vi "Main.vi"(8 "error in (no error)":errorcluster, 11 "ModuleAdmin":refnum<class "ModuleAdmin.lvclass">) -> ()   [LabVIEW 2018, in "SyncModule.lvlib"]
uses:
  SyncModule.lvlib
  <userlib>/NIST/ModuleAdminLib/ModuleAdmin/ModuleAdmin.lvclass
  C:/Program Files (x86)/National Instruments/LabVIEW 2018/user.lib/NIST/ModuleAdminLib/ModuleAdminBase/ModuleAdminBase.lvclass
  SyncPlugins/SyncPluginBase/SyncPluginBase.lvclass
  C:/Program Files (x86)/National Instruments/LabVIEW 2018/user.lib/NIST/BaseClasses/BasePlugin_class/BasePlugin.lvclass
  PublicAPI/Arguments/Requests/clStopArgument.ctl
  SyncPlugins/SyncPluginBase/SyncPluginBase.lvclass/SyncPluginBase.ctl
  <userlib>/NIST/BaseClasses/BasePlugin_class/BasePlugin.lvclass/BasePlugin.ctl
  <userlib>/NIST/ModuleAdminLib/ModuleAdmin/ModuleAdmin.lvclass/ModuleAdmin.ctl
  SyncPlugins/SyncPluginBase/Typedefs/clEnaTrigTmstmp.ctl
  SyncPlugins/SyncPluginBase/Typedefs/clGetTrigTmstmp.ctl
  SyncPlugins/SyncPluginBase/Typedefs/clTimedTrigger.ctl
  <vilib>/Utility/error.llb/DialogType.ctl
  SyncPlugins/SyncPluginBase/Accessors/Read PPSTime.vi
  <userlib>/NIST/BaseClasses/BasePlugin_class/Accessors/Read PluginIniFilePath.vi
  <userlib>/NIST/ModuleAdminLib/ModuleAdmin/Accessors/Read ShowPanel_.vi
  <userlib>/NIST/ModuleAdminLib/ModuleAdmin/Accessors/Write ShowPanel_.vi
  <userlib>/NIST/BaseClasses/BasePlugin_class/Accessors/Write PluginIniFilePath.vi
  SyncPlugins/SyncPluginBase/Accessors/Write LostLock.vi
  <userlib>/NIST/ModuleAdminLib/ModuleAdmin/Accessors/Read CloneRegRef.vi
  <extravilib>/ChannelInstances/Tag-bool/Read With Abort.vi
  <extravilib>/ChannelInstances/Tag-bool/Write With Abort.vi
  <extravilib>/ChannelInstances/Tag-bool/Instantiate.vi
  <extravilib>/ChannelInstances/Tag-bool/EndpointRead.vi
  SyncPlugins/SyncPluginBase/Accessors/Read Clocks.vi
  SyncPlugins/SyncPluginBase/Accessors/Write Clocks.vi
  <vilib>/Utility/error.llb/Error Cluster From Error Code.vi
  <extravilib>/ChannelInstances/Tag-bool/Endpoint.vi
  <vilib>/ErrorRing/Error Ring.xnode
  <userlib>/NIST/ModuleAdminLib/CloneRegistration/CloneRegistration.lvclass
  <userlib>/NIST/BaseClasses/Object_class/BaseObject.lvclass
  <userlib>/NIST/ModuleAdminLib/ModuleAdmin.lvlib
  <extravilib>/ChannelInstances/Tag-bool.lvlib
panel:
  out "Data Acquistion Loop State":string
  out "Class Name":string
  out "INI File Name":string
  in  "btReset":bool
  out "PPSTime":timestamp
  out "Time Ref Offset (ns)":dbl format="%#_12f"
  out "Locked":bool
  out "error out":errorcluster
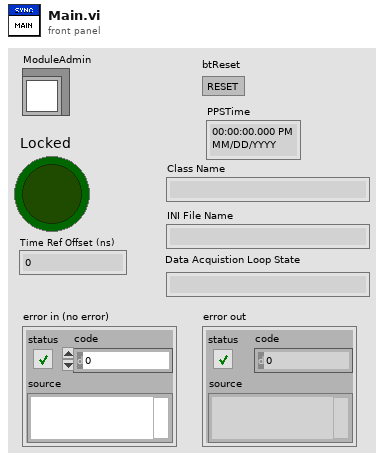
[diagram p1: front panel]
types:
  T1 = typedef "SyncModule.lvlib/clRequestEvents.ctl" = cluster{"StopRequest":refnum<user-event>, "PathToINI":refnum<user-event>, " LoadPlugin":refnum<user-event>, "ShowPanel":refnum<user-event>, "LockToUTC":refnum<user-event>, "TriggerTime":refnum<user-event>, "ConfigDlg":refnum<user-event>, "Initialize":refnum<user-event>, "ConfigClk":refnum<user-event>, "ConfigTrig":refnum<user-event>, "SoftwareTrig":refnum<user-event>, "TimedTrig":refnum<user-event>, "EnaTrigTmstmp":refnum<user-event>, "GetTrigTmstmp":refnum<user-event>, "GetInfo":refnum<user-event>, "GetClockProperties":refnum<user-event>, "SetClockProperties":refnum<user-event>}
  T2 = typedef "SyncModule.lvlib/clBroadcastEvents.ctl" = cluster{"DidInit":refnum<user-event>, "StatusUpdate":refnum<user-event>, "ErrorReport":refnum<user-event>, "DidStop":refnum<user-event>, "PathToINI":refnum<user-event>, "TriggerTime":refnum<user-event>, "LockStatus":refnum<user-event>, "Info":refnum<user-event>, "ClockProperties":refnum<user-event>, "New TimeRefOffset Val":refnum<user-event>}
  T3 = typedef "SyncModule.lvlib/clStopArgument.ctl" = cluster{"Exit via Stop Module Req?":bool, "Wait for Module to stop?":bool, "ModuleAdmin":refnum<class "ModuleAdmin.lvclass">}
  T4 = enum32{"Invalid", "Standard", "Closed", "Hidden", "Minimized", "Maximized"}
  T5 = typedef "SyncPlugins.lvlib/SyncPluginBase.lvclass/clEnaTrigTmstmp.ctl" = cluster{"TriggerName":string, "Enable":bool}
  T6 = typedef "SyncPlugins.lvlib/SyncPluginBase.lvclass/clGetTrigTmstmp.ctl" = cluster{"TriggerName":string, "Timeout (s)":dbl}
  T7 = typedef "SyncPlugins.lvlib/SyncPluginBase.lvclass/clTimedTrigger.ctl" = cluster{"TriggerName":string, "Time after next UTC Second":dbl, "Trigger Duration":dbl, "Edge":enum16{"Rising", "Falling"}}
  T8 = cluster{"seconds since 1Jan1904":timestamp, "Time Ref Offset (ns)":dbl, "Lock":bool}
  T9 = typedef "Tag-bool.lvlib/))Channel.ctl" = refnum<queue>
  T10 = typedef "DialogType.ctl" = u16
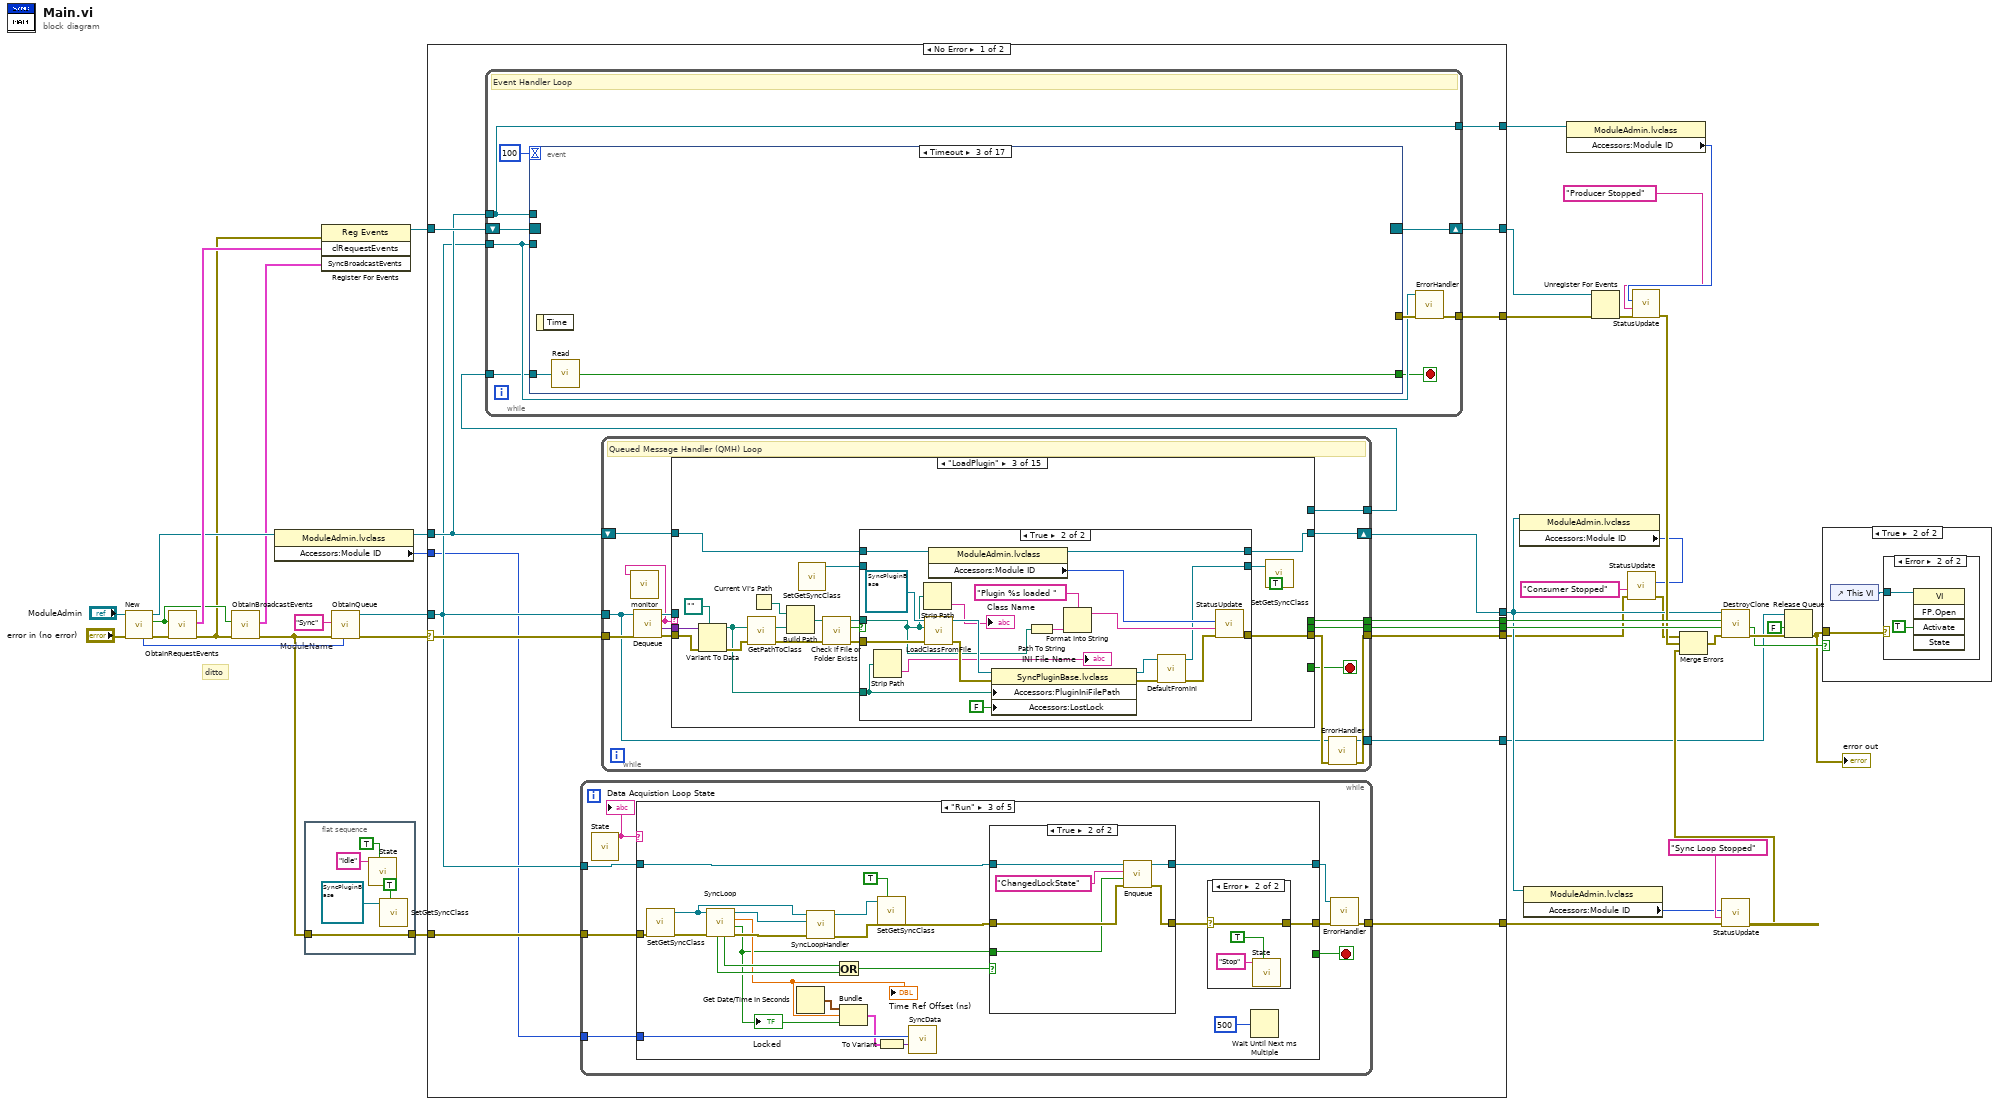
[diagram p0: block diagram]
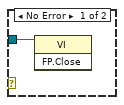
[diagram p3: hidden frame]
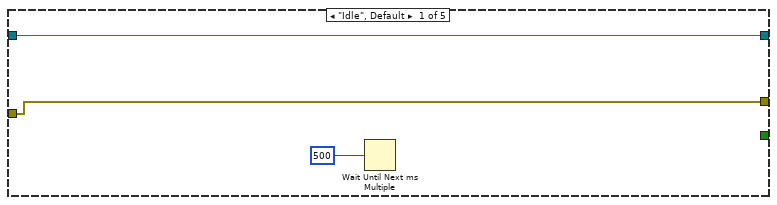
[diagram p4: hidden frame]
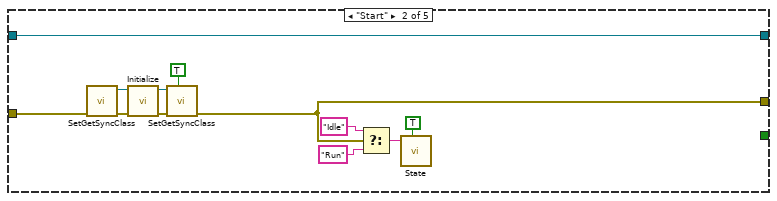
[diagram p5: hidden frame]
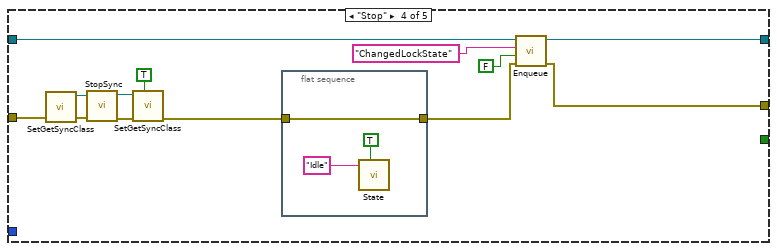
[diagram p8: hidden frame]
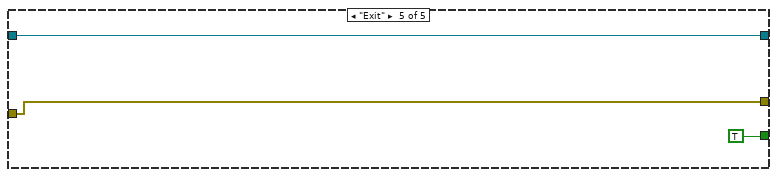
[diagram p9: hidden frame]
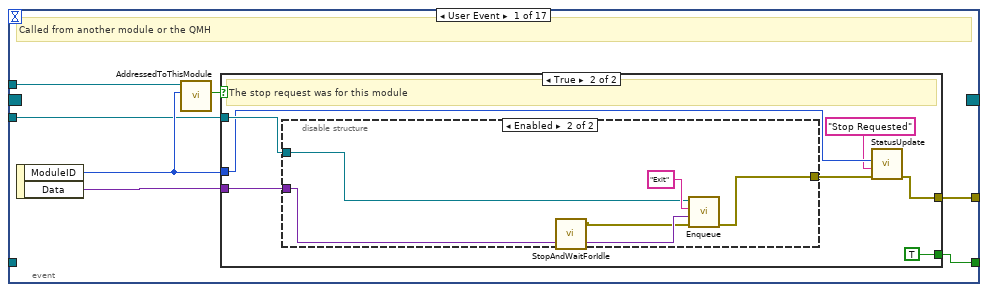
[diagram p10: hidden frame]
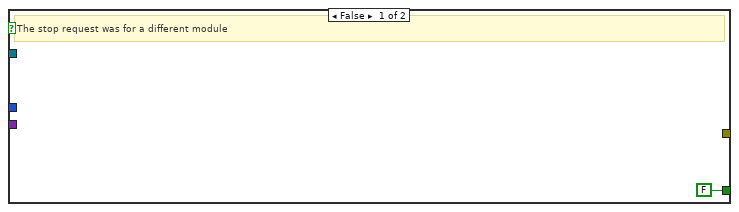
[diagram p11: hidden frame]
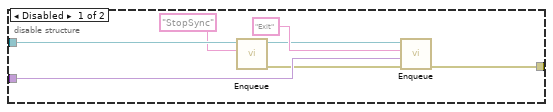
[diagram p12: hidden frame]
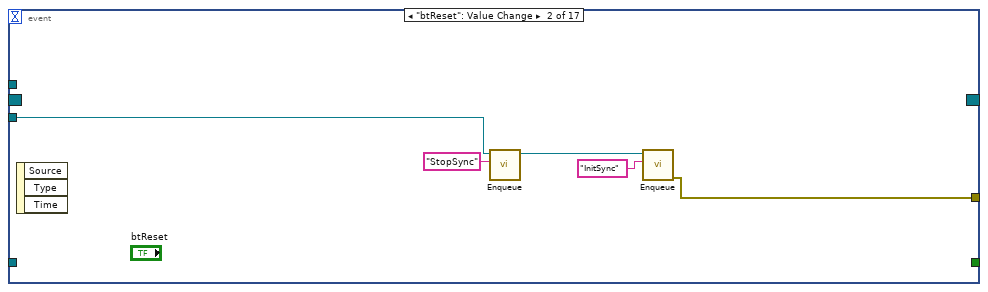
[diagram p13: hidden frame]
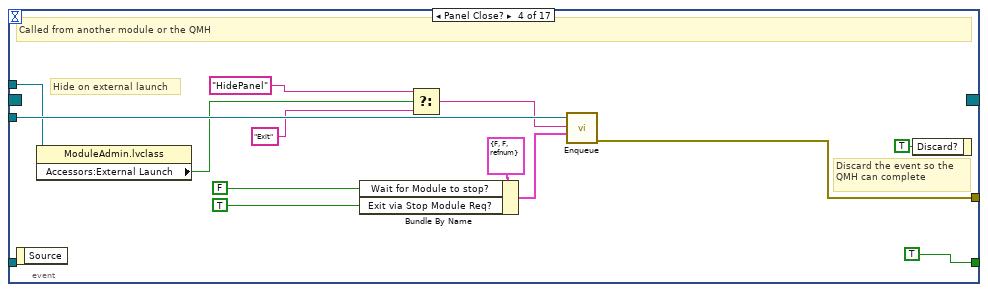
[diagram p14: hidden frame]
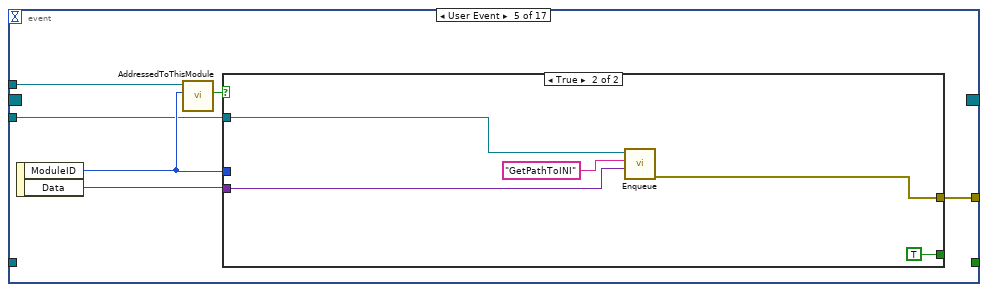
[diagram p15: hidden frame]
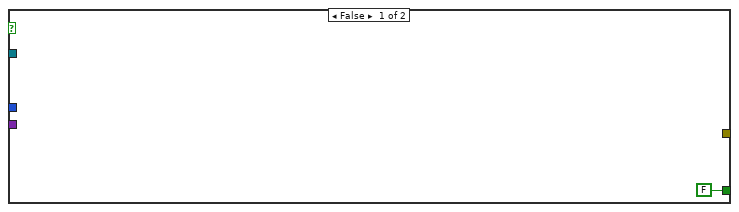
[diagram p16: hidden frame]
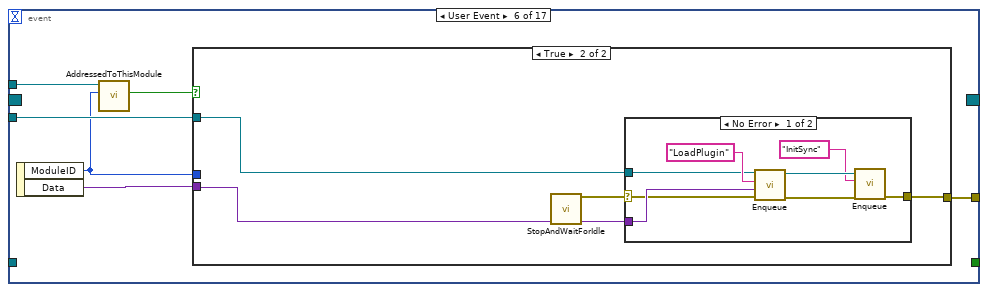
[diagram p17: hidden frame]
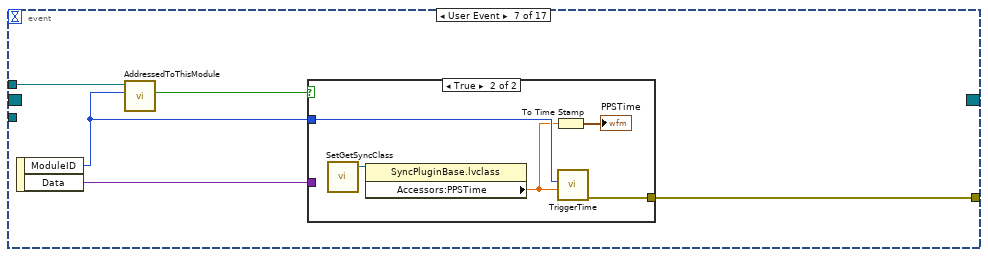
[diagram p20: hidden frame]
diagram:
  w7 = "Sync"  # ModuleName
  # "ditto"
  n1 = call <userlib>:"New.vi"("error in (no error)"="error in (no error)", "ModuleAdmin"="ModuleAdmin") -> ("error out"=w40:errorcluster, "First?"=w35:bool, "ModuleAdmin"=w36:refnum<class "ModuleAdmin.lvclass">, "Module ID"=w8:i32)  [unwired: 4 in, 2 out]
  n2 = call "ObtainRequestEvents.vi"("error in (no error)"=w40, "CreateNew (F)"=w35) -> ("error out"=w34:errorcluster, "clRequestEvents"=w39:T1)  [unwired: 8 in]
  n3 = call "ObtainBroadcastEvents.vi"("error in (no error)"=w34, "CreateNew? (F)"=w35) -> ("error out"=w6:errorcluster, "SyncBroadcastEvents"=w33:T2)  [unwired: 8 in]
  n4 = property class="ModuleAdmin.lvclass"(reference=w36) -> (reference out=w2:refnum<class "ModuleAdmin.lvclass">, "Accessors:Module ID"=w1:i32)  [unwired: 1 in, 1 out]
  n5 = flat-sequence {
    tunnel: w6 -> [w44]
    tunnel: [w44] -> w5
    frame #0 {
      n6 = call "State.vi"("Set (f)"=TRUE, "State"="Idle") -> ()  [unwired: 9 in, 1 out]
      n7 = call "SetGetSyncClass.vi"("Set? (f)"=TRUE, "SyncPluginBase in"=refnum<class "SyncPluginBase.lvclass"> refnum ("MyPlugins.lvlib:MyPluginsBase.lvclass")) -> ()  [unwired: 9 in, 1 out]
    }
  }
  n8 = register-events(error in=w34, w39, w33) -> (reference out=w32:refnum<event-registration>)  [unwired: 1 in, 1 out]
  n9 = call "ObtainQueue.vi"("ModuleNumber"=w8, "error in (no error)"=w6, "ModuleName"=w7) -> ("error out"=w38:errorcluster, "MessageQueue"=w37:refnum<queue>)  [unwired: 7 in]
  n10 = case shown="No Error" w38 {
    selector: w38 -> [w62 w627]
    tunnel: w37 -> [w54 w619]
    tunnel: w2 -> [w59 w620]
    tunnel: [w61 w625] -> w11
    tunnel: w32 -> [w60 w621]
    tunnel: [w58 w624] -> w13
    tunnel: [w57 _] -> w26
    tunnel: [w56 _] -> w27
    tunnel: [w55 _] -> w28
    tunnel: [w53 _] -> w18
    tunnel: [w52 w621] -> w29
    tunnel: [w51 w620] -> w24
    tunnel: w5 -> [w50 _]
    tunnel: [w49 w619] -> w3
    tunnel: w1 -> [w47 _]
    frame No Error {
      n11 = while {
        tunnel: w54 -> [w69]
        tunnel: [w70] -> w53
        tunnel: w50 -> [w66]
        tunnel: w47 -> [w63]
        stop <- w64 stop-if-true
        n12 = call "State.vi"() -> ("State"=w65:string)  [unwired: 11 in]
        "Data Acquistion Loop State" <- w65
        n13 = case shown="\"Run\"" w65 {
          tunnel: w69 -> [w73 w79 w100 w122 w131]
          tunnel: [w73 w79 w104 w121 w131] -> w68
          tunnel: [w72 w74 w94 w117 w132] -> w67
          tunnel: w66 -> [w72 w77 w96 w124 w132]
          tunnel: [_ _ _ _ TRUE] -> w64
          tunnel: w63 -> [_ _ w89 _ _]
          frame "Idle", Default {
            n14 = Wait Until Next ms Multiple(millisecond multiple=500) -> ()  [unwired: 1 out]
          }
          frame "Start" {
            n15 = call "SetGetSyncClass.vi"() -> ("SyncPluginBase out"=w76:refnum<class "SyncPluginBase.lvclass">)  [unwired: 11 in]
            n16 = call-dynamic "Initialize.vi"("error in (no error)"=w77, "SyncPluginBase in"=w76) -> ("error out"=w74:errorcluster, "SyncPluginBase out"=w75:refnum<class "SyncPluginBase.lvclass">)  [unwired: 8 in]
            n17 = call "SetGetSyncClass.vi"("Set? (f)"=TRUE, "SyncPluginBase in"=w75) -> ()  [unwired: 9 in, 1 out]
            n18 = Select(t="Idle", s=w74, f="Run") -> (s? t:f=w80:string)
            n19 = call "State.vi"("Set (f)"=TRUE, "State"=w80) -> ()  [unwired: 9 in, 1 out]
          }
          frame "Run" {
            n20 = call "SetGetSyncClass.vi"() -> ("SyncPluginBase out"=w92:refnum<class "SyncPluginBase.lvclass">)  [unwired: 11 in]
            n21 = call-dynamic "SyncLoop.vi"("error in (no error)"=w96, "SyncPluginBase in"=w92) -> ("error out"=w98:errorcluster, "Lock"=w87:bool, "Time Ref Offset (ns)"=w88:dbl, "SyncPluginBase out"=w99:refnum<class "SyncPluginBase.lvclass">, "LostLock"=w102:bool, "ObtainLock"=w101:bool)  [unwired: 4 in]
            "Locked" <- w87
            "Time Ref Offset (ns)" <- w88
            n22 = Get Date/Time In Seconds() -> (seconds since 1Jan1904=w86:timestamp)
            n23 = call-dynamic "SyncLoopHandler.vi"("error in (no error)"=w98, "LoopProperties"=w99, "SyncPluginBase in"=w92) -> ("error out"=w97:errorcluster, "SyncPluginBase out"=w91:refnum<class "SyncPluginBase.lvclass">)  [unwired: 7 in]
            n24 = Or(x=w102, y=w101) -> (x .or. y?=w103:bool)
            n25 = Bundle("seconds since 1Jan1904"=w86, "Time Ref Offset (ns)"=w88, "Lock"=w87) -> (w85:T8)  [unwired: 1 in]
            n26 = call "SetGetSyncClass.vi"("Set? (f)"=TRUE, "SyncPluginBase in"=w91) -> ()  [unwired: 9 in, 1 out]
            n27 = To Variant(anything=w85) -> (Variant=w84:variant)
            n28 = call "SyncData.vi"("Data"=w84, "ModuleID"=w89) -> ()  [unwired: 9 in, 1 out]
            n29 = case shown="True" w103 {
              tunnel: w100 -> [w110 w116]
              tunnel: [w110 w115] -> w104
              tunnel: [w109 w113] -> w95
              tunnel: w97 -> [w109 w112]
              tunnel: w87 -> [_ w111]
              frame False {
              }
              frame True {
                n30 = call "Enqueue.vi"("error in (no error)"=w112, "Message Data"=w111, "Message"="ChangedLockState", "MessageQueue"=w116) -> ("error out"=w113:errorcluster, "MessageQueue"=w115:refnum<queue>)  [unwired: 6 in]
              }
            }
            n31 = case shown="Error" w95 {
              selector: w95 -> [w105 w108]
              tunnel: [w105 w108] -> w94
              frame No Error {
              }
              frame Error {
                n32 = call "State.vi"("Set (f)"=TRUE, "State"="Stop") -> ()  [unwired: 9 in, 1 out]
              }
            }
            n33 = Wait Until Next ms Multiple(millisecond multiple=u32 500) -> ()  [unwired: 1 out]
          }
          frame "Stop" {
            n34 = call "SetGetSyncClass.vi"() -> ("SyncPluginBase out"=w127:refnum<class "SyncPluginBase.lvclass">)  [unwired: 11 in]
            n35 = call-dynamic "StopSync.vi"("error in (no error)"=w124, "SyncPluginBase in"=w127) -> ("error out"=w123:errorcluster, "SyncPluginBase out"=w125:refnum<class "SyncPluginBase.lvclass">)  [unwired: 8 in]
            n36 = call "SetGetSyncClass.vi"("Set? (f)"=TRUE, "SyncPluginBase in"=w125) -> ()  [unwired: 9 in, 1 out]
            n37 = flat-sequence {
              tunnel: w123 -> [w128]
              tunnel: [w128] -> w118
              frame #0 {
                n38 = call "State.vi"("Set (f)"=TRUE, "State"="Idle") -> ()  [unwired: 9 in, 1 out]
              }
            }
            n39 = call "Enqueue.vi"("error in (no error)"=w118, "Message Data"=FALSE, "Message"="ChangedLockState", "MessageQueue"=w122) -> ("error out"=w117:errorcluster, "MessageQueue"=w121:refnum<queue>)  [unwired: 6 in]
          }
          frame "Exit" {
          }
        }
        n40 = call "ErrorHandler.vi"("error in (no error)"=w67, "MessageQueue"=w68) -> ("error out"=w70:errorcluster)  [unwired: 8 in, 1 out]
      }
      n41 = while {
        tunnel: w54 -> [w372]
        tunnel: w62 -> [w380]
        tunnel: [w374] -> w61
        tunnel: [w376] -> w57
        tunnel: [w375] -> w56
        shift-right: [w371] -> w58
        shift-left: w59 -> [w377]
        tunnel: [w367] -> w49
        tunnel: [w366] -> w48
        stop <- w370 stop-if-true
        # "Queued Message Handler (QMH) Loop"
        n42 = call "Dequeue.vi"("error in (no error)"=w380, "MessageQueue"=w372) -> ("error out"=w379:errorcluster, "Message Data"=w378:variant, "Message"=w368:string, "MessageQueue"=w369:refnum<queue>)  [unwired: 6 in]
        n43 = call "monitor.vi"("Command"=w368) -> ()  [unwired: 11 in]
        n44 = case shown="\"LoadPlugin\"" w368 {
          selector: w368 -> [_ _ _ _ _ _ _ _ _ _ _ _ _ _ w607]
          tunnel: [_ _ _ _ _ _ _ _ _ _ _ _ w587 _ _] -> w370
          tunnel: w377 -> [w401 w417 w426 w477 w484 w494 w505 w513 w534 w549 w558 w572 w582 w589 w610]
          tunnel: [w390 w410 w427 w478 w485 w489 w501 w514 w535 w538 w559 w564 w586 w590 w606] -> w373
          tunnel: w379 -> [_ w420 w436 w471 w482 w490 w507 w516 w526 w546 w553 w571 w577 w598 _]
          tunnel: w378 -> [_ w419 w438 _ _ _ w506 _ w525 w547 w554 w570 w581 w597 _]
          tunnel: [_ _ _ _ _ _ _ _ _ _ _ _ w584 _ _] -> w376
          tunnel: [_ _ _ _ _ _ _ _ _ _ _ _ w583 _ _] -> w375
          tunnel: [w382 w416 w425 w476 w480 w493 w503 w512 w533 w540 w557 w566 w580 w588 w604] -> w371
          tunnel: w369 -> [_ _ _ _ _ _ _ _ _ _ _ _ _ _ _]
          tunnel: [_ _ _ _ _ _ _ _ _ _ _ _ w573 _ _] -> w366
          frame "Initialize" {
            # "Initialize is always called after ObtainQueue.vi is run"
            n45 = property class="ModuleAdmin.lvclass"(reference=w401) -> (reference out=w387:refnum<class "ModuleAdmin.lvclass">, error out=w398:errorcluster, "Accessors:Module ID"=w389:i32, "Accessors:ShowPanel_"=w385:bool, "Accessors:External Launch"=w384:bool, "Accessors:ModuleName"=w386:string)  [unwired: 1 in]
            n46 = Compound Arithmetic op=OR(w385, invert w384) -> (w383:bool)
            n47 = property on="Locked" class="Bool (strict)"("Value"=FALSE ("Locked")) -> ()  [unwired: 2 in, 2 out]
            n48 = Select(t=T4."Standard" ("Front Panel Window:State"), s=w383, f=T4."Hidden" ("Front Panel Window:State")) -> (s? t:f=w394:T4)
            n49 = invoke class="VI" method="FP.Open"(error in=w398, "State"=w394) -> (error out=w397:errorcluster)  [unwired: 3 in, 4 out]
            n50 = call <userlib>:"ModuleName.vi"("Name"=w386, "ModuleID"=w389) -> ("ModuleName"=w393:string)  [unwired: 9 in]
            n51 = property class="VI"(error in=w397, "Front Panel.Title"=w393) -> (reference out=w400:refnum<vi>, error out=w399:errorcluster)  [unwired: 1 in]
            n52 = invoke class="VI" method="FP.Center"(reference=w400, error in=w399) -> (error out=w388:errorcluster)  [unwired: 1 in, 2 out]
            n53 = case shown="True" w384 {
              tunnel: [w402 w408] -> w391
              tunnel: [w403 w405] -> w382
              tunnel: w388 -> [w402 w407]
              tunnel: w387 -> [w403 w404]
              frame False {
              }
              frame True {
                n54 = call <userlib>:"WaitOnModuleSync.vi"("error in (no error)"=w407, "ModuleAdmin"=w404) -> ("error out"=w409:errorcluster, "ModuleAdmin"=w406:refnum<class "ModuleAdmin.lvclass">)  [unwired: 8 in]
                n55 = call <userlib>:"WaitOnEventSync.vi"("error in (no error)"=w409, "ModuleAdmin"=w406) -> ("error out"=w408:errorcluster, "ModuleAdmin"=w405:refnum<class "ModuleAdmin.lvclass">)  [unwired: 8 in]
              }
            }
            n56 = call "DidInit.vi"("Init?"=TRUE, "error in (no error)"=w391, "ModuleAdmin"=w382) -> ("error out"=w390:errorcluster)  [unwired: 8 in]
          }
          frame "ShowPanel" {
            n57 = Variant To Data(error in=w420, type=TRUE, Variant=w419) -> (data=w412:bool, error out=w415:errorcluster)
            n58 = Select(t=T4."Standard" ("Front Panel Window:State"), s=w412, f=T4."Hidden" ("Front Panel Window:State")) -> (s? t:f=w411:T4)
            n59 = property class="VI"(error in=w415, "FP.State"=w411) -> (error out=w410:errorcluster)  [unwired: 1 in, 1 out]
            n60 = property class="ModuleAdmin.lvclass"(reference=w417, "Accessors:ShowPanel_"=w412) -> (reference out=w416:refnum<class "ModuleAdmin.lvclass">)  [unwired: 1 in, 1 out]
          }
          frame "LoadPlugin" {
            n61 = Variant To Data(error in=w436, type=path "", Variant=w438) -> (data=w424:path, error out=w435:errorcluster)
            n62 = call <userlib>:"GetPathToClass.vi"("error in (no error)"=w435, "configuration file path"=w424) -> ("error IO"=w431:errorcluster, "PathToClass"=w434:path)  [unwired: 8 in]
            n63 = Current VI's Path() -> (path=w433:path)
            n64 = Build Path(base path=w433, name or relative path=w434) -> (appended path=w432:path)
            n65 = call "SetGetSyncClass.vi"() -> ("SyncPluginBase out"=w423:refnum<class "SyncPluginBase.lvclass">)  [unwired: 11 in]
            n66 = call <vilib>:"Check if File or Folder Exists.vi"("error in (no error)"=w431, "path"=w432) -> ("error out"=w428:errorcluster, "file or folder exists?"=w430:bool, "dup path"=w429:path)  [unwired: 7 in]
            n67 = case shown="True" w430 {
              tunnel: w429 -> [w442 w452]
              tunnel: w428 -> [_ w470]
              tunnel: [w441 w456] -> w427
              tunnel: w426 -> [w439 w465]
              tunnel: w423 -> [w440 _]
              tunnel: [w440 w457] -> w422
              tunnel: w424 -> [_ w454]
              tunnel: [w439 w461] -> w425
              frame False {
                n68 = Path To String(path=w442) -> (string=w443:string)
                n69 = xnode "Error Ring"("parameter 0"=w443) -> ("error out"=w441:errorcluster)
              }
              frame True {
                n70 = Strip Path(path=w454) -> (name=→"INI File Name":string)  [unwired: 1 out]
                n71 = Strip Path(path=w452) -> (name=→"Class Name":string)  [unwired: 1 out]
                n72 = call-dynamic "LoadClassFromFile.vi"("error in (no error)"=w470, "class path"=w452, "reference in"=refnum<class "SyncPluginBase.lvclass"> refnum ("MyPlugins.lvlib:MyPluginsBase.lvclass")) -> ("error out"=w462:errorcluster, "reference out"=w463:refnum<class "SyncPluginBase.lvclass">)  [unwired: 7 in]
                n73 = property class="ModuleAdmin.lvclass"(reference=w465) -> (reference out=w461:refnum<class "ModuleAdmin.lvclass">, "Accessors:Module ID"=w464:i32)  [unwired: 1 in, 1 out]
                n74 = property class="SyncPluginBase.lvclass"(reference=w463, error in=w462, "Accessors:PluginIniFilePath"=w454, "Accessors:LostLock"=FALSE ("LostLock")) -> (reference out=w458:refnum<class "SyncPluginBase.lvclass">, error out=w460:errorcluster)
                n75 = Path To String(path=w452) -> (string=w467:string)
                n76 = Format Into String(format string="Plugin %s loaded ", w467) -> (resulting string=w466:string)  [unwired: 2 in, 1 out]
                n77 = call-dynamic "DefaultFromIni.vi"("error in (no error)"=w460, "SyncPlugin"=w458) -> ("error out"=w459:errorcluster, "SyncPlugin"=w457:refnum<class "SyncPluginBase.lvclass">)  [unwired: 8 in]
                n78 = call "StatusUpdate.vi"("error in (no error)"=w459, "Status"=w466, "ModuleID"=w464) -> ("error out"=w456:errorcluster)  [unwired: 8 in]
              }
            }
            n79 = call "SetGetSyncClass.vi"("Set? (f)"=TRUE, "SyncPluginBase in"=w422) -> ()  [unwired: 9 in, 1 out]
          }
          frame "InitSync" {
            n80 = property class="ModuleAdmin.lvclass"(reference=w477) -> (reference out=w476:refnum<class "ModuleAdmin.lvclass">, "Accessors:Module ID"=w475:i32)  [unwired: 1 in, 1 out]
            n81 = call "State.vi"("Set (f)"=TRUE, "State"="Start") -> ()  [unwired: 9 in, 1 out]
            n82 = call "StatusUpdate.vi"("error in (no error)"=w471, "Status"="Initializing Sync", "ModuleID"=w475) -> ("error out"=w478:errorcluster)  [unwired: 8 in]
          }
          frame "GetPathToINI" {
            n83 = call "SetGetSyncClass.vi"() -> ("SyncPluginBase out"=w479:refnum<class "SyncPluginBase.lvclass">)  [unwired: 11 in]
            n84 = property class="SyncPluginBase.lvclass"(reference=w479, error in=w482) -> (error out=w481:errorcluster, "Accessors:PluginIniFilePath"=w483:path)  [unwired: 1 out]
            n85 = property class="ModuleAdmin.lvclass"(reference=w484) -> (reference out=w480:refnum<class "ModuleAdmin.lvclass">, "Accessors:Module ID"=w486:i32)  [unwired: 1 in, 1 out]
            n86 = call "PathToINIBroadcast.vi"("error in (no error)"=w481, "PathToINI"=w483, "ModuleID"=w486) -> ("error out"=w485:errorcluster)  [unwired: 8 in]
          }
          frame "StopSync" {
            n87 = property class="ModuleAdmin.lvclass"(reference=w494) -> (reference out=w493:refnum<class "ModuleAdmin.lvclass">, "Accessors:Module ID"=w491:i32)  [unwired: 1 in, 1 out]
            n88 = call "StatusUpdate.vi"("error in (no error)"=w490, "Status"="Stopping Sync", "ModuleID"=w491) -> ("error out"=w489:errorcluster)  [unwired: 8 in]
            n89 = call "State.vi"("Set (f)"=TRUE, "State"="Stop") -> ()  [unwired: 9 in, 1 out]
          }
          frame "ChangedLockState" {
            n90 = property class="ModuleAdmin.lvclass"(reference=w505) -> (reference out=w503:refnum<class "ModuleAdmin.lvclass">, "Accessors:Module ID"=w495:i32)  [unwired: 1 in, 1 out]
            n91 = Variant To Data(error in=w507, type=TRUE, Variant=w506) -> (data=w498:bool, error out=w504:errorcluster)
            n92 = Select(t="Obtained Lock", s=w498, f="Lost Lock") -> (s? t:f=w499:string)
            n93 = call "StatusUpdate.vi"("error in (no error)"=w504, "Status"=w499, "ModuleID"=w495) -> ("error out"=w502:errorcluster)  [unwired: 8 in]
            n94 = call "LockStatus.vi"("error in (no error)"=w502, "Locked?"=w498, "ModuleID"=w495) -> ("error out"=w501:errorcluster)  [unwired: 8 in]
          }
          frame "SoftwareTrig" {
            n95 = call "SetGetSyncClass.vi"() -> ("SyncPluginBase out"=w515:refnum<class "SyncPluginBase.lvclass">)  [unwired: 11 in]
            n96 = call-dynamic "SoftwareTrigger.vi"("error in (no error)"=w516, "SyncPluginBase in"=w515) -> ("error out"=w509:errorcluster)  [unwired: 8 in, 1 out]
            n97 = property class="ModuleAdmin.lvclass"(reference=w513, error in=w509) -> (reference out=w512:refnum<class "ModuleAdmin.lvclass">, error out=w508:errorcluster, "Accessors:Module ID"=w511:i32)
            n98 = call "StatusUpdate.vi"("error in (no error)"=w508, "Status"="Software Trigger", "ModuleID"=w511) -> ("error out"=w514:errorcluster)  [unwired: 8 in]
          }
          frame "EnaTrigTmstmp" {
            n99 = Variant To Data(error in=w526, type=T5 {"TriggerName"="", "Enable"=FALSE} ("clEnaTrigTmstmp"), Variant=w525) -> (data=w518:T5, error out=w519:errorcluster)
            n100 = call "SetGetSyncClass.vi"() -> ("SyncPluginBase out"=w523:refnum<class "SyncPluginBase.lvclass">)  [unwired: 11 in]
            n101 = Unbundle By Name(w518) -> ("Enable"=w517:bool)
            n102 = call-dynamic "EnaTrigTmstmp.vi"("error in (no error)"=w519, "clEnaTrigTmstmp"=w518, "SyncPluginBase in"=w523) -> ("error out"=w520:errorcluster, "SyncPluginBase out"=w522:refnum<class "SyncPluginBase.lvclass">)  [unwired: 7 in]
            n103 = call "SetGetSyncClass.vi"("Set? (f)"=TRUE, "SyncPluginBase in"=w522) -> ()  [unwired: 9 in, 1 out]
            n104 = property class="ModuleAdmin.lvclass"(reference=w534) -> (reference out=w533:refnum<class "ModuleAdmin.lvclass">, "Accessors:Module ID"=w532:i32)  [unwired: 1 in, 1 out]
            n105 = Select(t="Enabled", s=w517, f="Disabled") -> (s? t:f=w528:string)
            n106 = Concatenate Strings("Trig Timestamp " ("Status"), w528) -> (w527:string)
            n107 = call "StatusUpdate.vi"("error in (no error)"=w520, "Status"=w527, "ModuleID"=w532) -> ("error out"=w535:errorcluster)  [unwired: 8 in]
          }
          frame "GetTrigTmstmp" {
            n108 = Variant To Data(error in=w546, type=T6 {"TriggerName"="", "Timeout (s)"=1.0} ("clEnaTrigTmstmp"), Variant=w547) -> (data=w544:T6, error out=w545:errorcluster)
            n109 = property class="ModuleAdmin.lvclass"(reference=w549) -> (reference out=w540:refnum<class "ModuleAdmin.lvclass">, "Accessors:Module ID"=w537:i32)  [unwired: 1 in, 1 out]
            n110 = call "SetGetSyncClass.vi"() -> ("SyncPluginBase out"=w543:refnum<class "SyncPluginBase.lvclass">)  [unwired: 11 in]
            n111 = call-dynamic "GetTrigTmstmp.vi"("error in (no error)"=w545, "TriggerName"=w544, "SyncPluginBase in"=w543) -> ("error out"=w542:errorcluster, "Timestamp"=w541:dbl)  [unwired: 6 in, 1 out]
            n112 = call "TriggerTime.vi"("error in (no error)"=w542, "TriggerTime"=w541, "ModuleID"=w537) -> ("error out"=w539:errorcluster)  [unwired: 8 in]
            n113 = call "StatusUpdate.vi"("error in (no error)"=w539, "Status"="TriggerTime Bdcst", "ModuleID"=w537) -> ("error out"=w538:errorcluster)  [unwired: 8 in]
          }
          frame "TimedTrig" {
            n114 = property class="ModuleAdmin.lvclass"(reference=w558) -> (reference out=w557:refnum<class "ModuleAdmin.lvclass">, "Accessors:Module ID"=w556:i32)  [unwired: 1 in, 1 out]
            n115 = Variant To Data(error in=w553, type=T7 {"TriggerName"="", "Time after next UTC Second"=0.0, "Trigger Duration"=0.1, "Edge"=enum."Rising"} ("clTimedTrigger"), Variant=w554) -> (data=w551:T7, error out=w552:errorcluster)
            n116 = call "SetGetSyncClass.vi"() -> ("SyncPluginBase out"=w561:refnum<class "SyncPluginBase.lvclass">)  [unwired: 11 in]
            n117 = call-dynamic "TimedTrigger.vi"("error in (no error)"=w552, "Time after next UTC Second"=w551, "SyncPluginBase in"=w561) -> ("error out"=w560:errorcluster)  [unwired: 7 in, 1 out]
            n118 = call "StatusUpdate.vi"("error in (no error)"=w560, "Status"="Timed Trigger Enabled", "ModuleID"=w556) -> ("error out"=w559:errorcluster)  [unwired: 8 in]
          }
          frame "GetInfo" {
            n119 = property class="ModuleAdmin.lvclass"(reference=w572) -> (reference out=w566:refnum<class "ModuleAdmin.lvclass">, "Accessors:Module ID"=w562:i32)  [unwired: 1 in, 1 out]
            n120 = call "SetGetSyncClass.vi"() -> ("SyncPluginBase out"=w569:refnum<class "SyncPluginBase.lvclass">)  [unwired: 11 in]
            n121 = call-dynamic "GetInfo.vi"("error in (no error)"=w571, "Parameter"=w570, "SyncPluginBase in"=w569) -> ("error out"=w568:errorcluster, "Info"=w567:string[])  [unwired: 6 in, 1 out]
            n122 = call "Info.vi"("error in (no error)"=w568, "Info"=w567, "ModuleID"=w562) -> ("error out"=w565:errorcluster)  [unwired: 8 in]
            n123 = call "StatusUpdate.vi"("error in (no error)"=w565, "Status"="SyncInfo Bdcst", "ModuleID"=w562) -> ("error out"=w564:errorcluster)  [unwired: 8 in]
          }
          frame "Exit" {
            w587 = TRUE
            # "Called by the StopRequest event handler case"
            n124 = property class="ModuleAdmin.lvclass"(reference=w582) -> (reference out=w580:refnum<class "ModuleAdmin.lvclass">, "Accessors:Module ID"=w579:i32)  [unwired: 1 in, 1 out]
            n125 = call "StatusUpdate.vi"("error in (no error)"=w577, "Status"="Exiting", "ModuleID"=w579) -> ("error out"=w574:errorcluster)  [unwired: 8 in]
            n126 = call "State.vi"("Set (f)"=TRUE, "State"="Exit") -> ()  [unwired: 9 in, 1 out]
            n127 = control-ref of="This VI"() -> (w585:refnum<vi>)
            n128 = call "HandleExit.vi"("error in (no error)"=w574, "VI Refnum"=w585, "StopArgument"=w581, "ModuleAdmin"=w580) -> ("error out"=w586:errorcluster, "Exit via Stop Module Req?"=w583:bool, "WaitForStop?"=w584:bool)  [unwired: 5 in]
            n129 = call <extravilib>:"Write.vi"("element"=w587) -> ("channel"=w573:T9)  [unwired: 1 out]
          }
          frame "Error" {
            n130 = property class="ModuleAdmin.lvclass"(reference=w589) -> (reference out=w588:refnum<class "ModuleAdmin.lvclass">, "Accessors:External Launch"=w593:bool, "Accessors:Module ID"=w591:i32)  [unwired: 1 in, 1 out]
            n131 = Variant To Data(error in=w598, type=errorcluster {"status"=FALSE, "code"=0, "source"=""} ("error constant"), Variant=w597) -> (data=w592:errorcluster, error out=w595:errorcluster)
            n132 = call "ReportError.vi"("error in (no error)"=w595, "ErrorReported"=w592, "ModuleID"=w591) -> ("error out"=w594:errorcluster)  [unwired: 8 in]
            n133 = case shown="False" w593 {
              tunnel: w594 -> [w602 w603]
              tunnel: w592 -> [w601 _]
              tunnel: [w600 w603] -> w590
              tunnel: w589 -> [w599 _]
              frame False {
                # "Todo:  Add an event to ask the user\nIf the module should stop or continue"
                # "Stand alone: now, force an exit"
                n134 = call <vilib>:"Simple Error Handler.vi"("error in (no error)"=w601) -> ()  [unwired: 4 in, 5 out]
                n135 = call "StopRequest.vi"("error in (no error)"=w602, "ModuleAdmin"=w599) -> ("error out"=w600:errorcluster)  [unwired: 8 in, 1 out]
              }
              frame True {
                # "Externally launched modules only broadcast the error msg"
              }
            }
          }
          frame Default {
            # "Called only if a message was queued and no QMH case was created"
            n136 = property class="ModuleAdmin.lvclass"(reference=w610) -> (reference out=w604:refnum<class "ModuleAdmin.lvclass">, "Accessors:Module ID"=w609:i32, "Accessors:ModuleName"=w605:string)  [unwired: 1 in, 1 out]
            n137 = call <userlib>:"ModuleName.vi"("Name"=w605, "ModuleID"=w609) -> ("ModuleName"=w608:string)  [unwired: 9 in]
            n138 = xnode "Error Ring"("parameter 0"=w607, "parameter 1"=w608) -> ("error out"=w606:errorcluster)
          }
        }
        n139 = call "ErrorHandler.vi"("error in (no error)"=w373, "MessageQueue"=w372) -> ("error out"=w374:errorcluster, "MessageQueue"=w367:refnum<queue>)  [unwired: 8 in]
      }
      n140 = while {
        tunnel: w54 -> [w140]
        shift-right: [w138] -> w52
        shift-left: w60 -> [w139]
        tunnel: w59 -> [w136]
        tunnel: [w141] -> w55
        tunnel: [w136] -> w51
        tunnel: w48 -> [w134]
        stop <- w137 stop-if-true
        # "Event Handler Loop"
        n141 = event shown="[2] Timeout" {
          selector: w139 -> [_ _ _ _ _ _ _ _ _ _ _ _ _ _ _ _ _]
          dyn-events: [_ _ _ _ _ _ _ _ _ _ _ _ _ _ _ _ _] -> w138
          timeout: 100 -> [_ _ _ _ _ _ _ _ _ _ _ _ _ _ _ _ _]
          tunnel: w140 -> [w146 w171 _ w189 w192 w205 _ _ w240 w250 w280 w290 w300 w310 w320 w332 w342]
          tunnel: [w145 _ w175 TRUE _ _ _ _ _ _ _ _ _ _ _ _ _] -> w137
          tunnel: w136 -> [w149 _ _ w183 w191 w207 w225 w235 w244 w254 w284 w294 w304 w314 w324 w334 w344]
          tunnel: [w144 w174 _ w187 w190 w206 w222 w232 w241 w251 w281 w291 w301 w311 w321 w330 w340] -> w142
          tunnel: w134 -> [_ _ w176 _ _ _ _ _ _ _ _ _ _ _ _ _ _]
          event User Event {
            # "Called from another module or the QMH"
            n142 = event-data() -> ("ModuleID"=w147:i32, "Data"=w143:variant)  [unwired: 1 in]
            n143 = call <userlib>:"AddressedToThisModule.vi"("ModuleID"=w147, "ModuleAdmin In"=w149) -> ("AddressedToThisInstance?"=w148:bool)  [unwired: 7 in, 2 out]
            n144 = case shown="True" w148 {
              tunnel: w147 -> [_ w153]
              tunnel: w146 -> [_ w157]
              tunnel: [FALSE TRUE] -> w145
              tunnel: [_ w151] -> w144
              tunnel: w143 -> [_ w155]
              frame False {
                # "The stop request was for a different module"
              }
              frame True {
                # "The stop request was for this module"
                n145 = disable-structure shown="Enabled" {
                  disable-tunnel: w157 -> [w164 w165]
                  disable-tunnel: w155 -> [w162 w168]
                  disable-tunnel: [w158 w169] -> w154
                  frame Disabled {
                    n146 = call "Enqueue.vi"("Message"="StopSync", "MessageQueue"=w164) -> ("error out"=w161:errorcluster, "MessageQueue"=w159:refnum<queue>)  [unwired: 8 in]
                    n147 = call "Enqueue.vi"("error in (no error)"=w161, "Message Data"=w162, "Message"="Exit", "MessageQueue"=w159) -> ("error out"=w158:errorcluster)  [unwired: 6 in, 1 out]
                  }
                  frame Enabled {
                    n148 = call "StopAndWaitForIdle.vi"() -> ("error out"=w166:errorcluster)  [unwired: 10 in, 1 out]
                    n149 = call "Enqueue.vi"("error in (no error)"=w166, "Message Data"=w168, "Message"="Exit", "MessageQueue"=w165) -> ("error out"=w169:errorcluster)  [unwired: 6 in, 1 out]
                  }
                }
                n150 = call "StatusUpdate.vi"("error in (no error)"=w154, "Status"="Stop Requested", "ModuleID"=w153) -> ("error out"=w151:errorcluster)  [unwired: 8 in]
              }
            }
          }
          event "btReset": Value Change {
            n151 = event-data() -> ()  [unwired: 1 in, 3 out]
            n152 = call "Enqueue.vi"("Message"="StopSync", "MessageQueue"=w171) -> ("MessageQueue"=w172:refnum<queue>)  [unwired: 8 in, 1 out]
            n153 = call "Enqueue.vi"("Message"="InitSync", "MessageQueue"=w172) -> ("error out"=w174:errorcluster)  [unwired: 8 in, 1 out]
          }
          event Timeout {
            n154 = event-data() -> ()  [unwired: 1 in, 1 out]
            n155 = call <extravilib>:"Read.vi"("channel"=w176) -> ("element"=w175:bool)  [unwired: 1 in, 1 out]
          }
          event Panel Close? {
            # "Hide on external launch"
            # "Discard the event so the QMH can complete"
            # "Called from another module or the QMH"
            n156 = event-data() -> ()  [unwired: 1 in, 1 out]
            n157 = property class="ModuleAdmin.lvclass"(reference=w183) -> ("Accessors:External Launch"=w178:bool)  [unwired: 1 in, 2 out]
            n158 = Bundle By Name(cluster=T3 {"Exit via Stop Module Req?"=FALSE, "Wait for Module to stop?"=FALSE, "ModuleAdmin"=refnum} ("Stop Argument"), "Wait for Module to stop?"=FALSE, "Exit via Stop Module Req?"=TRUE) -> (w184:T3)
            n159 = Select(t="HidePanel", s=w178, f="Exit" ("Message")) -> (s? t:f=w180:string)
            n160 = call "Enqueue.vi"("Message Data"=w184, "Message"=w180, "MessageQueue"=w189) -> ("error out"=w187:errorcluster)  [unwired: 7 in, 1 out]
            n161 = event-data("Discard?"=TRUE) -> ()  [unwired: 1 in, 1 out]
          }
          event User Event {
            n162 = event-data() -> ("ModuleID"=w193:i32, "Data"=w194:variant)  [unwired: 1 in]
            n163 = call <userlib>:"AddressedToThisModule.vi"("ModuleID"=w193, "ModuleAdmin In"=w191) -> ("AddressedToThisInstance?"=w195:bool)  [unwired: 7 in, 2 out]
            n164 = case shown="True" w195 {
              tunnel: w193 -> [_ _]
              tunnel: w192 -> [_ w201]
              tunnel: [FALSE TRUE] -> _
              tunnel: [_ w199] -> w190
              tunnel: w194 -> [_ w197]
              frame False {
                # "The stop request was for a different module"
              }
              frame True {
                # "The stop request was for this module"
                n165 = call "Enqueue.vi"("Message Data"=w197, "Message"="GetPathToINI", "MessageQueue"=w201) -> ("error out"=w199:errorcluster)  [unwired: 7 in, 1 out]
              }
            }
          }
          event User Event {
            n166 = event-data() -> ("ModuleID"=w203:i32, "Data"=w204:variant)  [unwired: 1 in]
            n167 = call <userlib>:"AddressedToThisModule.vi"("ModuleID"=w203, "ModuleAdmin In"=w207) -> ("AddressedToThisInstance?"=w202:bool)  [unwired: 7 in, 2 out]
            n168 = case shown="True" w202 {
              tunnel: [_ w211] -> w206
              tunnel: w205 -> [_ w208]
              tunnel: w204 -> [_ w210]
              tunnel: w203 -> [_ _]
              frame False {
              }
              frame True {
                n169 = call "StopAndWaitForIdle.vi"() -> ("error out"=w209:errorcluster)  [unwired: 10 in, 1 out]
                n170 = case shown="No Error" w209 {
                  selector: w209 -> [w213 w220]
                  tunnel: [w215 w220] -> w211
                  tunnel: w210 -> [w214 _]
                  tunnel: w208 -> [w212 _]
                  frame No Error {
                    n171 = call "Enqueue.vi"("error in (no error)"=w213, "Message Data"=w214, "Message"="LoadPlugin", "MessageQueue"=w212) -> ("error out"=w218:errorcluster, "MessageQueue"=w217:refnum<queue>)  [unwired: 6 in]
                    n172 = call "Enqueue.vi"("error in (no error)"=w218, "Message"="InitSync", "MessageQueue"=w217) -> ("error out"=w215:errorcluster)  [unwired: 7 in, 1 out]
                  }
                  frame Error {
                  }
                }
              }
            }
          }
          event User Event {
            n173 = event-data() -> ("ModuleID"=w221:i32, "Data"=w223:variant)  [unwired: 1 in]
            n174 = call <userlib>:"AddressedToThisModule.vi"("ModuleID"=w221, "ModuleAdmin In"=w225) -> ("AddressedToThisInstance?"=w224:bool)  [unwired: 7 in, 2 out]
            n175 = case shown="True" w224 {
              tunnel: w223 -> [_ _]
              tunnel: [_ w228] -> w222
              tunnel: w221 -> [_ w229]
              frame False {
              }
              frame True {
                n176 = call "SetGetSyncClass.vi"() -> ("SyncPluginBase out"=w230:refnum<class "SyncPluginBase.lvclass">)  [unwired: 11 in]
                n177 = property class="SyncPluginBase.lvclass"(reference=w230) -> ("Accessors:PPSTime"=w227:dbl)  [unwired: 1 in, 2 out]
                n178 = To Time Stamp(1:w227) -> (0:→"PPSTime":timestamp)
                n179 = call "TriggerTime.vi"("TriggerTime"=w227, "ModuleID"=w229) -> ("error out"=w228:errorcluster)  [unwired: 9 in]
              }
            }
          }
          event User Event {
            n180 = event-data() -> ("ModuleID"=w231:i32, "Data"=w233:variant)  [unwired: 1 in]
            n181 = call <userlib>:"AddressedToThisModule.vi"("ModuleID"=w231, "ModuleAdmin In"=w235) -> ("AddressedToThisInstance?"=w234:bool)  [unwired: 7 in, 2 out]
            n182 = case shown="True" w234 {
              tunnel: w233 -> [_ _]
              tunnel: [_ w238] -> w232
              tunnel: w231 -> [_ w236]
              frame False {
              }
              frame True {
                n183 = property on="Locked" class="Bool (strict)"() -> ("Value"=w237:bool)  [unwired: 2 in, 2 out]
                n184 = call "LockStatus.vi"("Locked?"=w237, "ModuleID"=w236) -> ("error out"=w238:errorcluster)  [unwired: 9 in]
              }
            }
          }
          event User Event {
            n185 = event-data() -> ("ModuleID"=w243:i32, "Data"=w239:variant)  [unwired: 1 in]
            n186 = call <userlib>:"AddressedToThisModule.vi"("ModuleID"=w243, "ModuleAdmin In"=w244) -> ("AddressedToThisInstance?"=w242:bool)  [unwired: 7 in, 2 out]
            n187 = case shown="True" w242 {
              tunnel: [_ w245] -> w241
              tunnel: w240 -> [_ w248]
              tunnel: w239 -> [_ w246]
              frame False {
              }
              frame True {
                n188 = call "Enqueue.vi"("Message Data"=w246, "Message"="ShowPanel", "MessageQueue"=w248) -> ("error out"=w245:errorcluster)  [unwired: 7 in, 1 out]
              }
            }
          }
          event User Event {
            n189 = event-data() -> ("ModuleID"=w253:i32, "Data"=w249:variant)  [unwired: 1 in]
            n190 = call <userlib>:"AddressedToThisModule.vi"("ModuleID"=w253, "ModuleAdmin In"=w254) -> ("AddressedToThisInstance?"=w252:bool)  [unwired: 7 in, 2 out]
            n191 = case shown="True" w252 {
              tunnel: [_ w256] -> w251
              tunnel: w250 -> [_ w257]
              tunnel: w249 -> [_ _]
              frame False {
              }
              frame True {
                n192 = call "SetGetSyncClass.vi"() -> ("SyncPluginBase out"=w260:refnum<class "SyncPluginBase.lvclass">)  [unwired: 11 in]
                n193 = call-dynamic "ConfigureDlg.vi"("SyncPluginBase in"=w260) -> ("error out"=w258:errorcluster, "Changed?"=w259:bool, "SyncPluginBase out"=w255:refnum<class "SyncPluginBase.lvclass">)  [unwired: 8 in]
                n194 = case shown="True" w259 {
                  tunnel: w258 -> [w261 w265]
                  tunnel: w257 -> [_ w263]
                  tunnel: [w261 w269] -> w256
                  tunnel: w255 -> [_ w268]
                  frame False {
                  }
                  frame True {
                    n195 = property class="SyncPluginBase.lvclass"(reference=w268, error in=w265) -> (error out=w264:errorcluster, "Accessors:PluginIniFilePath"=w267:path)  [unwired: 1 out]
                    n196 = To Variant(anything=w267) -> (Variant=w266:variant)
                    n197 = call "StopAndWaitForIdle.vi"("error in (no error)"=w264) -> ("error out"=w262:errorcluster)  [unwired: 9 in, 1 out]
                    n198 = case shown="No Error" w262 {
                      selector: w262 -> [w270 w278]
                      tunnel: [w277 w278] -> w269
                      tunnel: w266 -> [w272 _]
                      tunnel: w263 -> [w271 _]
                      frame No Error {
                        n199 = call "Enqueue.vi"("error in (no error)"=w270, "Message Data"=w272, "Message"="LoadPlugin", "MessageQueue"=w271) -> ("error out"=w274:errorcluster, "MessageQueue"=w273:refnum<queue>)  [unwired: 6 in]
                        n200 = call "Enqueue.vi"("error in (no error)"=w274, "Message"="InitSync", "MessageQueue"=w273) -> ("error out"=w277:errorcluster)  [unwired: 7 in, 1 out]
                      }
                      frame Error {
                      }
                    }
                  }
                }
              }
            }
          }
          event User Event {
            n201 = event-data() -> ("ModuleID"=w283:i32, "Data"=w279:variant)  [unwired: 1 in]
            n202 = call <userlib>:"AddressedToThisModule.vi"("ModuleID"=w283, "ModuleAdmin In"=w284) -> ("AddressedToThisInstance?"=w282:bool)  [unwired: 7 in, 2 out]
            n203 = case shown="True" w282 {
              tunnel: [_ w285] -> w281
              tunnel: w280 -> [_ w288]
              tunnel: w279 -> [_ w286]
              frame False {
              }
              frame True {
                n204 = call "Enqueue.vi"("Message Data"=w286, "Message"="SoftwareTrig", "MessageQueue"=w288) -> ("error out"=w285:errorcluster)  [unwired: 7 in, 1 out]
              }
            }
          }
          event User Event {
            n205 = event-data() -> ("ModuleID"=w293:i32, "Data"=w289:variant)  [unwired: 1 in]
            n206 = call <userlib>:"AddressedToThisModule.vi"("ModuleID"=w293, "ModuleAdmin In"=w294) -> ("AddressedToThisInstance?"=w292:bool)  [unwired: 7 in, 2 out]
            n207 = case shown="True" w292 {
              tunnel: [_ w295] -> w291
              tunnel: w290 -> [_ w298]
              tunnel: w289 -> [_ w296]
              frame False {
              }
              frame True {
                n208 = call "Enqueue.vi"("Message Data"=w296, "Message"="TimedTrig", "MessageQueue"=w298) -> ("error out"=w295:errorcluster)  [unwired: 7 in, 1 out]
              }
            }
          }
          event User Event {
            n209 = event-data() -> ("ModuleID"=w303:i32, "Data"=w299:variant)  [unwired: 1 in]
            n210 = call <userlib>:"AddressedToThisModule.vi"("ModuleID"=w303, "ModuleAdmin In"=w304) -> ("AddressedToThisInstance?"=w302:bool)  [unwired: 7 in, 2 out]
            n211 = case shown="True" w302 {
              tunnel: [_ w305] -> w301
              tunnel: w300 -> [_ w308]
              tunnel: w299 -> [_ w306]
              frame False {
              }
              frame True {
                n212 = call "Enqueue.vi"("Message Data"=w306, "Message"="EnaTrigTmstmp", "MessageQueue"=w308) -> ("error out"=w305:errorcluster)  [unwired: 7 in, 1 out]
              }
            }
          }
          event User Event {
            n213 = event-data() -> ("ModuleID"=w313:i32, "Data"=w309:variant)  [unwired: 1 in]
            n214 = call <userlib>:"AddressedToThisModule.vi"("ModuleID"=w313, "ModuleAdmin In"=w314) -> ("AddressedToThisInstance?"=w312:bool)  [unwired: 7 in, 2 out]
            n215 = case shown="True" w312 {
              tunnel: [_ w315] -> w311
              tunnel: w310 -> [_ w318]
              tunnel: w309 -> [_ w316]
              frame False {
              }
              frame True {
                n216 = call "Enqueue.vi"("Message Data"=w316, "Message"="GetTrigTmstmp", "MessageQueue"=w318) -> ("error out"=w315:errorcluster)  [unwired: 7 in, 1 out]
              }
            }
          }
          event User Event {
            n217 = event-data() -> ("ModuleID"=w323:i32, "Data"=w319:variant)  [unwired: 1 in]
            n218 = call <userlib>:"AddressedToThisModule.vi"("ModuleID"=w323, "ModuleAdmin In"=w324) -> ("AddressedToThisInstance?"=w322:bool)  [unwired: 7 in, 2 out]
            n219 = case shown="True" w322 {
              tunnel: [_ w325] -> w321
              tunnel: w320 -> [_ w328]
              tunnel: w319 -> [_ w326]
              frame False {
              }
              frame True {
                n220 = call "Enqueue.vi"("Message Data"=w326, "Message"="GetInfo", "MessageQueue"=w328) -> ("error out"=w325:errorcluster)  [unwired: 7 in, 1 out]
              }
            }
          }
          event User Event {
            n221 = event-data() -> ("ModuleID"=w329:i32, "Data"=w331:variant)  [unwired: 1 in]
            n222 = call <userlib>:"AddressedToThisModule.vi"("ModuleID"=w329, "ModuleAdmin In"=w334) -> ("AddressedToThisInstance?"=w333:bool)  [unwired: 7 in, 2 out]
            n223 = case shown="True" w333 {
              tunnel: w332 -> [_ _]
              tunnel: w331 -> [_ _]
              tunnel: [_ w338] -> w330
              tunnel: w329 -> [_ w335]
              frame False {
              }
              frame True {
                n224 = call "SetGetSyncClass.vi"() -> ("SyncPluginBase out"=w337:refnum<class "SyncPluginBase.lvclass">)  [unwired: 11 in]
                n225 = property class="SyncPluginBase.lvclass"(reference=w337) -> ("Accessors:Clocks"=w336:variant[])  [unwired: 1 in, 2 out]
                n226 = call "ClockProperties.vi"("ClockProperties"=w336, "ModuleID"=w335) -> ("error out"=w338:errorcluster)  [unwired: 9 in]
              }
            }
          }
          event User Event {
            n227 = event-data() -> ("ModuleID"=w339:i32, "Data"=w341:variant)  [unwired: 1 in]
            n228 = call <userlib>:"AddressedToThisModule.vi"("ModuleID"=w339, "ModuleAdmin In"=w344) -> ("AddressedToThisInstance?"=w343:bool)  [unwired: 7 in, 2 out]
            n229 = case shown="True" w343 {
              tunnel: w342 -> [_ w346]
              tunnel: w341 -> [_ w349]
              tunnel: [_ w345] -> w340
              tunnel: w339 -> [_ _]
              frame False {
              }
              frame True {
                n230 = Variant To Data(type=variant[] [], Variant=w349) -> (data=w347:variant[], error out=w350:errorcluster)  [unwired: 1 in]
                n231 = call "StopAndWaitForIdle.vi"("error in (no error)"=w350) -> ("error out"=w351:errorcluster)  [unwired: 9 in, 1 out]
                n232 = case shown="No Error" w351 {
                  selector: w351 -> [w359 w365]
                  tunnel: w347 -> [w358 _]
                  tunnel: w346 -> [w357 _]
                  tunnel: [w355 w365] -> w345
                  frame No Error {
                    n233 = call "SetGetSyncClass.vi"() -> ("SyncPluginBase out"=w360:refnum<class "SyncPluginBase.lvclass">)  [unwired: 11 in]
                    n234 = property class="SyncPluginBase.lvclass"(reference=w360, error in=w359, "Accessors:Clocks"=w358) -> (reference out=w354:refnum<class "SyncPluginBase.lvclass">, error out=w356:errorcluster)
                    n235 = call "SetGetSyncClass.vi"("Set? (f)"=TRUE, "SyncPluginBase in"=w354) -> ("SyncPluginBase out"=w352:refnum<class "SyncPluginBase.lvclass">)  [unwired: 9 in]
                    n236 = flat-sequence {
                      tunnel: [w364] -> w355
                      tunnel: w357 -> [w362]
                      tunnel: w356 -> [w361]
                      tunnel: w352 -> [_]
                      frame #0 {
                        n237 = call "Enqueue.vi"("error in (no error)"=w361, "Message"="InitSync", "MessageQueue"=w362) -> ("error out"=w364:errorcluster)  [unwired: 7 in, 1 out]
                      }
                    }
                  }
                  frame Error {
                  }
                }
              }
            }
          }
        }
        n238 = call "ErrorHandler.vi"("error in (no error)"=w142, "MessageQueue"=w140) -> ("error out"=w141:errorcluster)  [unwired: 8 in, 1 out]
      }
    }
    frame Error {
      n239 = property class="ModuleAdmin.lvclass"(reference=w620) -> (reference out=w624:refnum<class "ModuleAdmin.lvclass">, "Accessors:CloneRegRef"=w623:refnum<data-value>, "Accessors:Module ID"=w622:i32)  [unwired: 1 in, 1 out]
      n240 = call <userlib>:"Remove.vi"("Module ID"=w622, "CloneRegRef"=w623) -> ("error out"=w626:errorcluster)  [unwired: 7 in, 2 out]
      n241 = flat-sequence {
        tunnel: w627 -> [w630]
        tunnel: w626 -> [_]
        tunnel: [w628] -> w625
        frame #0 {
          w629 = T10 2 items=["no dialog", "OK message", "continue or stop message", "OK message + warnings", "continue/stop + warnings"] ("type of dialog (OK msg:1)")
          n242 = call <vilib>:"Simple Error Handler.vi"("type of dialog (OK msg:1)"=w629, "error in (no error)"=w630) -> ("error out"=w628:errorcluster)  [unwired: 3 in, 4 out]
        }
      }
    }
  }
  n243 = property class="ModuleAdmin.lvclass"(reference=w13) -> ("Accessors:Module ID"=w15:i32)  [unwired: 1 in, 2 out]
  n244 = property class="ModuleAdmin.lvclass"(reference=w13) -> ("Accessors:Module ID"=w12:i32)  [unwired: 1 in, 2 out]
  n245 = property class="ModuleAdmin.lvclass"(reference=w24) -> ("Accessors:Module ID"=w23:i32)  [unwired: 1 in, 2 out]
  n246 = Unregister For Events(event registration refnum=w29, error in=w28) -> (error out=w25:errorcluster)
  n247 = call "StatusUpdate.vi"("error in (no error)"=w11, "Status"="Consumer Stopped", "ModuleID"=w15) -> ("error out"=w10:errorcluster)  [unwired: 8 in]
  n248 = call "StatusUpdate.vi"("error in (no error)"=w25, "Status"="Producer Stopped", "ModuleID"=w23) -> ("error out"=w19:errorcluster)  [unwired: 8 in]
  n249 = call "StatusUpdate.vi"("error in (no error)"=w18, "Status"="Sync Loop Stopped", "ModuleID"=w12) -> ("error out"=w16:errorcluster)  [unwired: 8 in]
  n250 = Merge Errors(w10, w19, w16) -> (w20:errorcluster)
  n251 = call "DestroyClone.vi"("error in (no error)"=w20, "Exit via Stop Module Req?"=w27, "Wait for Module to stop?"=w26, "ModuleAdmin"=w13) -> ("error out"=w31:errorcluster, "External Launch"=w30:bool)  [unwired: 5 in, 1 out]
  n252 = Release Queue(queue=w3, force destroy? (F)=FALSE, error in (no error)=w31) -> (error out=w21:errorcluster)  [unwired: 2 out]
  "error out" <- w21
  n253 = case shown="True" w30 {
    tunnel: w21 -> [_ w632]
    frame False {
    }
    frame True {
      n254 = control-ref of="This VI"() -> (w631:refnum<vi>)
      n255 = case shown="Error" w632 {
        tunnel: w631 -> [w633 w634]
        frame No Error {
          n256 = invoke class="VI" method="FP.Close"(reference=w633) -> ()  [unwired: 2 in, 3 out]
        }
        frame Error {
          n257 = invoke class="VI" method="FP.Open"(reference=w634, "Activate"=TRUE ("Activate?")) -> ()  [unwired: 3 in, 5 out]
        }
      }
    }
  }
